vi "set_product_config.vi"(6 "timeout (25000ms)":i32=25000, 8 "error in (no error)":errorcluster, 9 "firmware SIV file":path, 10 "firmware image hex file":path, 11 "daemon reference in":refnum<k5>) -> (0 "error out":errorcluster, 2 "response":string, 3 "daemon reference out":refnum<k5>, 5 "command out":string="random")   [LabVIEW 2017]
doc: "<b>Command: </b>\"template\"\n\n<b>Description: </b> This command does something.\n\n<b>Parameters: </b> None\n____________________________________________\nDIPC 692 Daemon API 10.0.0.1\nSam Tee - Dyson Technology Ltd\nCopyright (c) 2024, Dyson Technology Ltd"
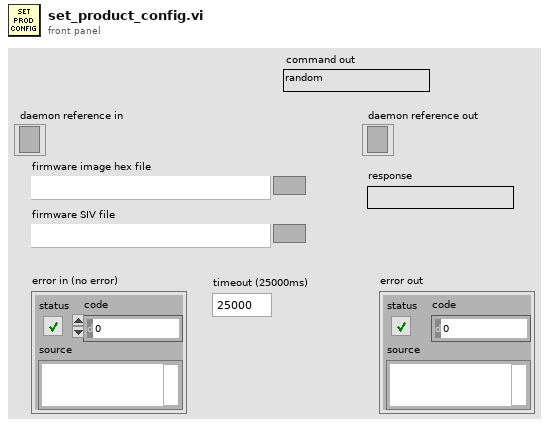
[diagram p1: front panel]
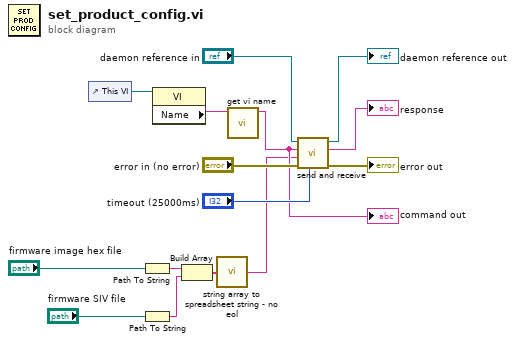
[diagram p0: block diagram]
diagram:
  n1 = control-ref of="This VI"() -> (w9:refnum<vi>)
  n2 = Path To String(path="firmware image hex file") -> (string=w4:string)
  n3 = Path To String(path="firmware SIV file") -> (string=w3:string)
  n4 = property class="VI"(reference=w9) -> ("Name"=w8:string)  [unwired: 1 in, 2 out]
  n5 = Build Array(w4, w3) -> (w2:string[])
  n6 = call "string array to spreadsheet string - no eol.vi"("string array"=w2) -> ("spreadsheet string - no eol"=w1:string)
  n7 = call "get vi name.vi"("library.lvlib:name.vi"=w8) -> ("vi name"=w7:string)  [unwired: 10 in]
  "command out" <- w7
  n8 = call "send and receive.vi"("timeout (25000ms)"="timeout (25000ms)", "error in (no error)"="error in (no error)", "data"=w1, "command"=w7, "daemon reference in"="daemon reference in") -> ("error out"=→"error out":errorcluster, "response"=→"response":string, "daemon reference out"=→"daemon reference out":refnum<k5>)  [unwired: 4 in]
